vi "DynamicCall.vi"() -> ()   [LabVIEW 2011]
panel:
  out "error out 3":errorcluster
  out "error out 2":errorcluster
  out "error out":errorcluster
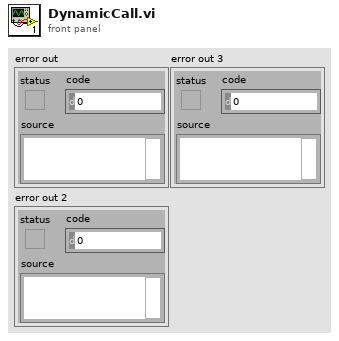
[diagram p1: front panel]
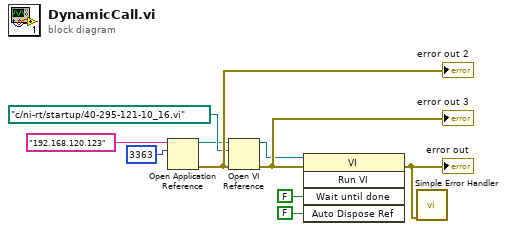
[diagram p0: block diagram]
diagram:
  n1 = Open Application Reference(10:u16 3363 ("port number or service name (3363)"), 11:"192.168.120.123" ("machine name (\"\":  open local reference)")) -> (0:w7:errorcluster, 3:w3:refnum<vi>)  [unwired: 2 in]
  "error out 2" <- w7
  n2 = Open VI Reference(application reference (local)=w3, vi path=path "c:/ni-rt/startup/40-295-121-10_16.vi", error in (no error)=w7) -> (vi reference=w1:refnum<vi>, error out=w10:errorcluster)  [unwired: 3 in]
  "error out 3" <- w10
  n3 = invoke class="VI" method="Run VI"(reference=w1, error in=w10, "Wait until done"=FALSE ("Wait Until Done"), "Auto Dispose Ref"=FALSE ("Auto Dispose Reference")) -> (error out=w2:errorcluster)  [unwired: 1 in, 4 out]
  "error out" <- w2
  n4 = call <vilib>:"Simple Error Handler.vi"("error in (no error)"=w2) -> ()  [unwired: 4 in, 5 out]
